vi "save data.vi"(6 "Procesar datos\nen Matlab":bool, 7 "iteration":i32, 8 "error in (no error)":errorcluster, 9 "Record":bool, 10 "data save DAQ":T1, 11 "queue":refnum<queue>) -> (0 "error out":errorcluster, 3 "queue out":refnum<queue>)   [LabVIEW 2013]
doc: "SubVI contain buffer to acquire data to simulation and/or DAQ system for save in temp file after analysis"
uses:
  bus to create file.ctl
  data simulation bus.ctl
  VoltElectrodo.ctl
  shell32.dll
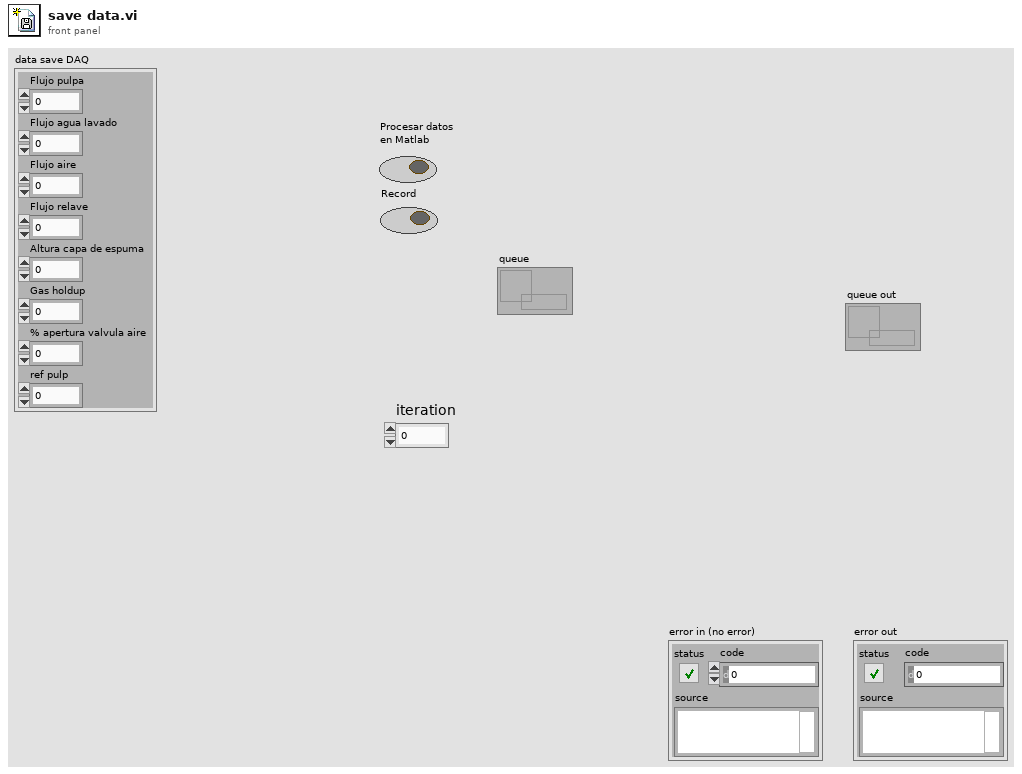
[diagram p1: front panel]
types:
  T1 = typedef "data simulation bus.ctl" = cluster{"Flujo pulpa ":dbl, "Flujo agua lavado":dbl, "Flujo aire":dbl, "Flujo relave":dbl, "Altura capa de espuma":dbl, "Gas holdup":dbl, "% apertura valvula aire":dbl, "ref pulp":dbl}
  T2 = typedef "bus to create file.ctl" = cluster{"data simulation":T1, "Time":dbl, "volt":T3}
  T3 = typedef "VoltElectrodo.ctl" = cluster{"V1":dbl, "V2":dbl, "V3":dbl, "V4":dbl, "V5":dbl, "V6":dbl, "V7":dbl, "V8":dbl}
  T4 = cluster{"hWndOwner":i32, "pidlRoot":i32, "pszDisplayName":i32, "lpszTitle":i32, "ulFlags":i32, "lpfn":i32, "lParam":i32, "iImage":i32}
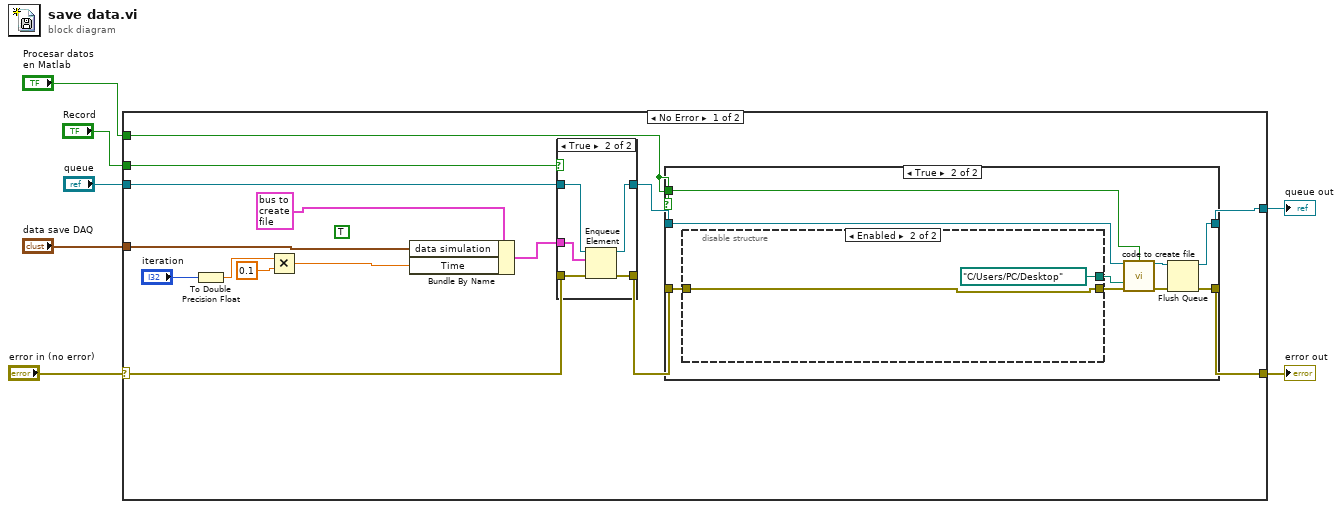
[diagram p0: block diagram]
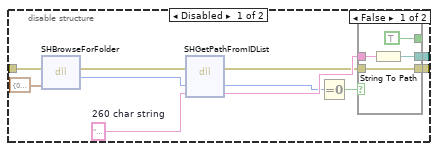
[diagram p3: hidden frame]
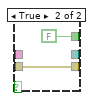
[diagram p4: hidden frame]
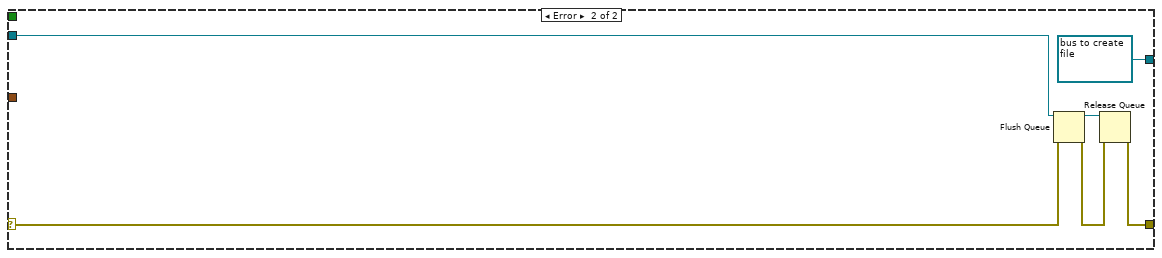
[diagram p6: hidden frame]
diagram:
  n1 = case shown="No Error" "error in (no error)" {
    selector: "error in (no error)" -> [w19 w65]
    tunnel: [w22 w62] -> w7
    tunnel: "Procesar datos\nen Matlab" -> [w8 _]
    tunnel: [w21 refnum<queue> refnum ("queue  out")] -> w5
    tunnel: "queue" -> [w20 w63]
    tunnel: "data save DAQ" -> [w14 _]
    tunnel: "Record" -> [w11 _]
    frame No Error {
      (unwired) TRUE
      n2 = To Double Precision Float(number="iteration") -> (double precision float=w12:dbl)
      n3 = Multiply(x=w12, y=0.1) -> (x*y=w15:dbl)
      n4 = Bundle By Name(cluster=T2 {"data simulation"={"Flujo pulpa "=0.0, "Flujo agua lavado"=0.0, "Flujo aire"=0.0, "Flujo relave"=0.0, "Altura capa de espuma"=0.0, "Gas holdup"=0.0, "% apertura valvula aire"=0.0, "ref pulp"=0.0}, "Time"=0.0, "volt"={"V1"=0.0, "V2"=0.0, "V3"=0.0, "V4"=0.0, "V5"=0.0, "V6"=0.0, "V7"=0.0, "V8"=0.0}}, "data simulation"=w14, "Time"=w15) -> (w18:T2)
      n5 = case shown="True" w11 {
        tunnel: [w53 w59] -> w9
        tunnel: w19 -> [w53 w58]
        tunnel: w20 -> [w54 w57]
        tunnel: w18 -> [_ w56]
        tunnel: [w54 w55] -> w10
        frame False {
        }
        frame True {
          n6 = Enqueue Element(queue=w57, element=w56, error in (no error)=w58) -> (queue out=w55:refnum<queue>, error out=w59:errorcluster)  [unwired: 1 in, 1 out]
        }
      }
      n7 = case shown="True" w8 {
        tunnel: w10 -> [w24 w33]
        tunnel: w9 -> [w23 w32]
        tunnel: [w23 w25] -> w22
        tunnel: [w24 w26] -> w21
        tunnel: w8 -> [_ w28]
        frame False {
        }
        frame True {
          n8 = disable-structure shown="Enabled" {
            disable-tunnel: w32 -> [w44 w51]
            disable-tunnel: [w43 path "C:/Users/PC/Desktop" ("Path")] -> w31
            disable-tunnel: [w42 w51] -> w29
            frame Disabled {
              w40 = "                                                                                                                                                                                                                                                      "  # 260 char string
              n9 = dll-call lib="shell32.dll" fn="SHBrowseForFolder"(error in=w44, "BROWSEINFO"=T4 {"hWndOwner"=0, "pidlRoot"=0, "pszDisplayName"=0, "lpszTitle"=0, "ulFlags"=1, "lpfn"=0, "lParam"=0, "iImage"=0}) -> (error out=w36:errorcluster, "PointerToIDList"=w37:i32)  [unwired: 3 in, 1 out]
              n10 = dll-call lib="shell32.dll" fn="SHGetPathFromIDList"(error in=w36, "PointerToIDList"=w37, "PathBuffer"=w40) -> (error out=w35:errorcluster, "PointerToIDList"=w34:i32, "PathBuffer"=w39:string)  [unwired: 3 in, 1 out]
              n11 = Equal To 0?(x=w34) -> (x = 0?=w38:bool)
              n12 = case shown="False" w38 {
                tunnel: w39 -> [w48 _]
                tunnel: [w47 w50] -> w42
                tunnel: w35 -> [w47 w50]
                tunnel: [w46 _] -> w43
                tunnel: [TRUE FALSE] -> _
                frame False {
                  n13 = String To Path(string=w48) -> (path=w46:path)
                }
                frame True {
                }
              }
            }
            frame Enabled {
            }
          }
          n14 = call "code to create file.vi"("queue"=w33, "Procesar datos en Matlab"=w28, "Path"=w31, "error in (no error)"=w29) -> ("queue  out"=w27:refnum<queue>, "error out"=w30:errorcluster)  [unwired: 10 in]
          n15 = Flush Queue(queue=w27, error in (no error)=w30) -> (queue out=w26:refnum<queue>, error out=w25:errorcluster)  [unwired: 1 out]
        }
      }
    }
    frame Error {
      n16 = Flush Queue(queue=w63, error in (no error)=w65) -> (queue out=w61:refnum<queue>, error out=w64:errorcluster)  [unwired: 1 out]
      n17 = Release Queue(queue=w61, error in (no error)=w64) -> (error out=w62:errorcluster)  [unwired: 1 in, 2 out]
    }
  }
  "error out" <- w7
  "queue out" <- w5
